vi "Get Section.vi"(11 "Mandatory Objects in":refnum<class "Mandatory Objects.lvclass">) -> (2 "Section":string, 3 "Mandatory Objects out":refnum<class "Mandatory Objects.lvclass">)   [LabVIEW 2024, in "EDS.lvlib" / "Mandatory Objects.lvclass"]
uses:
  Mandatory Objects.lvclass
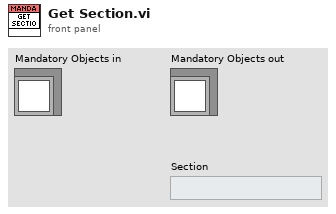
[diagram p1: front panel]
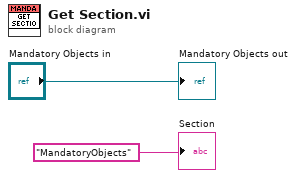
[diagram p0: block diagram]
diagram:
  "Mandatory Objects out" <- "Mandatory Objects in"
  "Section" <- "MandatoryObjects" ("Section")
